vi "CreatePrivateEvents.vi"(8 "error in (no error)":errorcluster, 11 "SMO.InstrumentDriver":refnum<class "SMO.InstrumentDriver.lvclass">) -> (0 "error out":errorcluster, 3 "SMO.InstrumentDriver out":refnum<class "SMO.InstrumentDriver.lvclass">)   [LabVIEW 2013, in "SMO.InstrumentDriver.lvclass"]
doc: "---------------------------------------------------------------\nJKI State Machine Objects™\nhttp://jki.net/state-machine-objects/\nCopyright (C) 2005-2015, JKI <info@jki.net>\nALL RIGHTS RESERVEDJKI State Machine Objects (SMO) 1.0.0.4\nJKI - JKI\nCopyright (c) 2015, JKI"
uses:
  SMO.InstrumentDriver.lvclass
  <vilib>/JKI/JKI SMO/SMO/SMO.lvclass
  SMO.InstrumentDriver.lvclass/SMO.InstrumentDriver.ctl
  Typedefs/WriteData.ctl
panel:
  # "For instructions on how to use the JKI State Machine Objects, examples and video tutorials, visit:\nhttp://jki.net/state-machine-objects/\n\nJKI State Machine Objects™\nhttp://jki.net/state-machine-objects/\nCopyright (C) 2005-2015, JKI <info@jki.net>\nALL RIGHTS RESERVED"
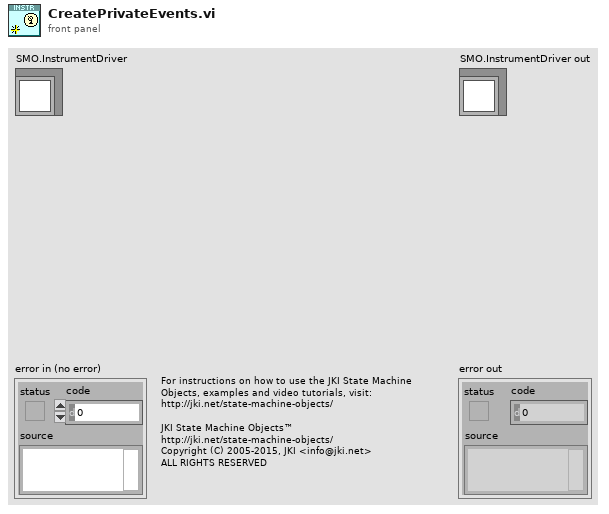
[diagram p1: front panel]
types:
  T1 = typedef "SMO.InstrumentDriver.lvclass/PrivateData--Ref.ctl" = refnum<data-value>
  T2 = typedef "SMO.InstrumentDriver.lvclass/WriteData.ctl" = dbl
  T3 = typedef "SMO.InstrumentDriver.lvclass/PrivateData--Cluster.ctl" = cluster{"Public Events":T4, "Private Events":T5}
  T4 = typedef "SMO.InstrumentDriver.lvclass/PublicEvents--Cluster.ctl" = cluster{"Value Changed":refnum<user-event>}
  T5 = typedef "SMO.InstrumentDriver.lvclass/PrivateEvents--Cluster.ctl" = cluster{"Write":refnum<user-event>}
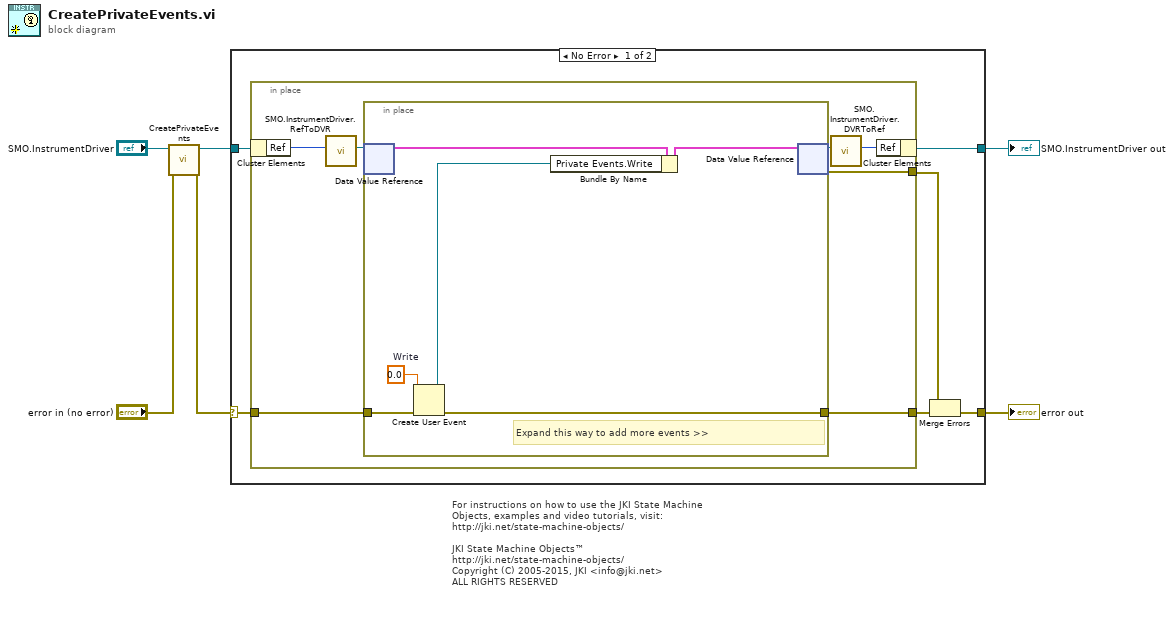
[diagram p0: block diagram]
diagram:
  # "For instructions on how to use the JKI State Machine Objects, examples and video tutorials, visit:\nhttp://jki.net/state-machine-objects/\n\nJKI State Machine Objects™\nhttp://jki.net/state-machine-objects/\nCopyright (C) 2005-2015, JKI <info@jki.net>\nALL RIGHTS RESERVED"
  n1 = call-parent "CreatePrivateEvents.vi"("error in (no error)"="error in (no error)", "SMO"="SMO.InstrumentDriver") -> ("error out"=w1:errorcluster, "SMO out"=w3:refnum<class "SMO.InstrumentDriver.lvclass">)  [unwired: 8 in]
  n2 = case shown="No Error" w1 {
    selector: w1 -> [w10 w27]
    tunnel: [w8 w27] -> w5
    tunnel: [w11 w26] -> w6
    tunnel: w3 -> [w12 w26]
    frame No Error {
      n3 = in-place {
        in-place-border: w10 -> [w19]
        in-place-border: [w16] -> w7
        in-place-border: [w15] -> w9
        n4 = in-place-cluster #1(w12) -> ("Ref"=w18:u32)
        n5 = call "SMO.InstrumentDriver.RefToDVR.vi"("Ref"=w18) -> ("Ref"=w14:T1)  [unwired: 10 in]
        n6 = in-place {
          in-place-border: w19 -> [w25]
          in-place-border: [w22] -> w16
          w21 = T2 0.0  # Write
          # "Expand this way to add more events >>"
          n7 = in-place-dvr #2(w14) -> (w24:T3)  [unwired: 1 out]
          n8 = Create User Event(user event datatype=w21, error in=w25) -> (user event=w20:refnum<user-event>, error out=w22:errorcluster)
          n9 = Bundle By Name(cluster=w24, "Private Events.Write"=w20) -> (w23:T3)
          n10 = in-place-dvr #2(w23) -> (w17:T1, w15:errorcluster)
        }
        n11 = call "SMO.InstrumentDriver.DVRToRef.vi"("Ref"=w17) -> ("Ref"=w13:u32)  [unwired: 10 in]
        n12 = in-place-cluster #1("Ref"=w13) -> (w11:refnum<class "SMO.InstrumentDriver.lvclass">)
      }
      n13 = Merge Errors(w9, w7) -> (w8:errorcluster)
    }
    frame Error {
    }
  }
  "error out" <- w5
  "SMO.InstrumentDriver out" <- w6
